vi "FTW-Endpoint-ZMQCore-SendMultipartMessage.vi"(0 "ØMQ Socket Pointer":u64 format="%016x", 5 "Multipart Message":string[](array[string]), 7 "Write Timeout":i32 format="%dmsec", 11 "error in":errorcluster) -> (4 "ØMQ Socket Pointer out":u64 format="%016x", 8 "Write Timed out?":bool, 15 "error out":errorcluster)   [LabVIEW 2012, in "FTW-Endpoint-ZMQ.lvclass"]
uses:
  FTW-Endpoint-ZMQ.lvclass
panel:
  # "Inputs"
  # "Outputs"
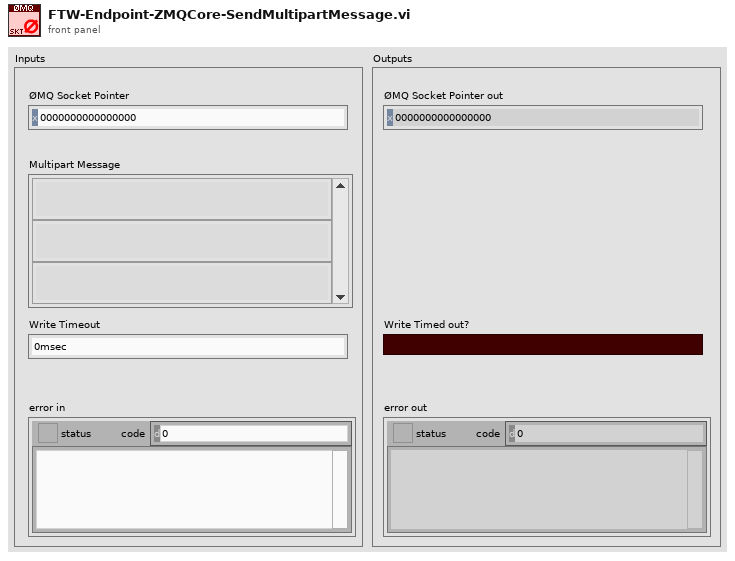
[diagram p1: front panel]
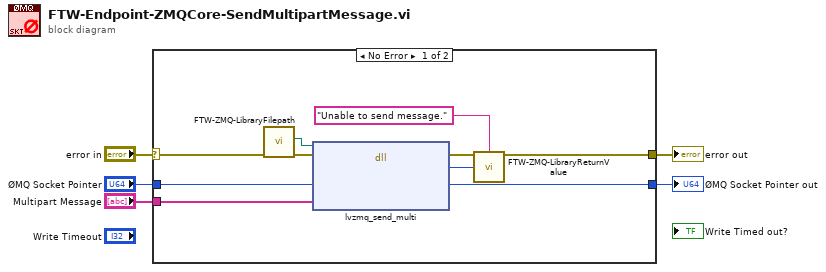
[diagram p0: block diagram]
diagram:
  n1 = case shown="No Error" "error in" {
    selector: "error in" -> [w13 w16]
    tunnel: "ØMQ Socket Pointer" -> [w7 w17]
    tunnel: "Multipart Message" -> [w15 _]
    tunnel: [w14 w16] -> w3
    tunnel: [w6 w17] -> w2
    frame No Error {
      n2 = call "FTW-ZMQ-LibraryFilepath.vi"("error in"=w13) -> ("error out"=w12:errorcluster, "FTW-ZMQ Library Filepath"=w11:path)  [unwired: 8 in, 1 out]
      n3 = dll-call lib="?" fn="lvzmq_send_multi" ("zmq_labview.dll:lvzmq_socket")(path in=w11, error in=w12, "Socket Pointer"=w7, "Multipart Message"=w15) -> (error out=w10:errorcluster, "Return Value"=w9:i32, "Socket Pointer"=w6:u64)  [unwired: 2 in, 1 out]
      n4 = call "FTW-ZMQ-LibraryReturnValue.vi"("error in"=w10, "Error Message"="Unable to send message.", "Return Value"=w9) -> ("error out"=w14:errorcluster)  [unwired: 12 in]
    }
    frame Error {
    }
  }
  "error out" <- w3
  "ØMQ Socket Pointer out" <- w2
